vi "FPGA_ADC_test.vi"() -> ()   [LabVIEW 2013]
uses:
  <vilib>/rvi/interface/nirviReadWriteControl/nirviReadWriteControl.xnode
  fpga-bitfile-ref.ctl
  <vilib>/rvi/interface/nirviCloseFPGA/nirviCloseFPGA.xnode
  FPGA Bitfiles/fpgabatch18_sbRIO9612RIO0_FPGAMAINlock-in_BbNldMosBaM.lvbitx
  <vilib>/rvi/errors/niLvFpgaMergeErrorWithErrorCode.vi
  <vilib>/rvi/errors/niLvFpgaAdjustHostInterfaceError.vi
  <vilib>/FPGAPlugInAG/sbRIO-9612/niLvFpga_Close_sbRIO-9612.vi
panel:
  out "data out":dbl[][](array[numeric])
  out "output cluster 2":T1
  out "output cluster":T2={"trig mode"=enum."ramp", "Nchannels"=0, "Navg"=0, "trig edge"=enum."falling", "trig input"=0, "Npts to read"=0, "Nchannels"=0, "clock divider"=0, "Data [i]"=0.0, "Configurations"=[0, 0, 0, 0, 0, 0, 0, 0, 0, 0, 0, 0, 0, 0, 0, 0, 0, 0, 0, 0, 0, 0, 0, 0, 0, 0, 0, 0, 0, 0, 0, 0]}
  in  "IP Address":string="192.168.137.11"
  in  "Inst_parameter":T3={"Kind"=17, "Strings"=["ADC", "192.168.137.11", "V0;V1", "V;V", "1.0;1.0", "0;1", "10;10", "RSE;RSE"], "uint64s"=[2, 250000, 1, 1, 0, 0, 1], "Doubles"=[1.0], "DAQmx take out list"=[]}
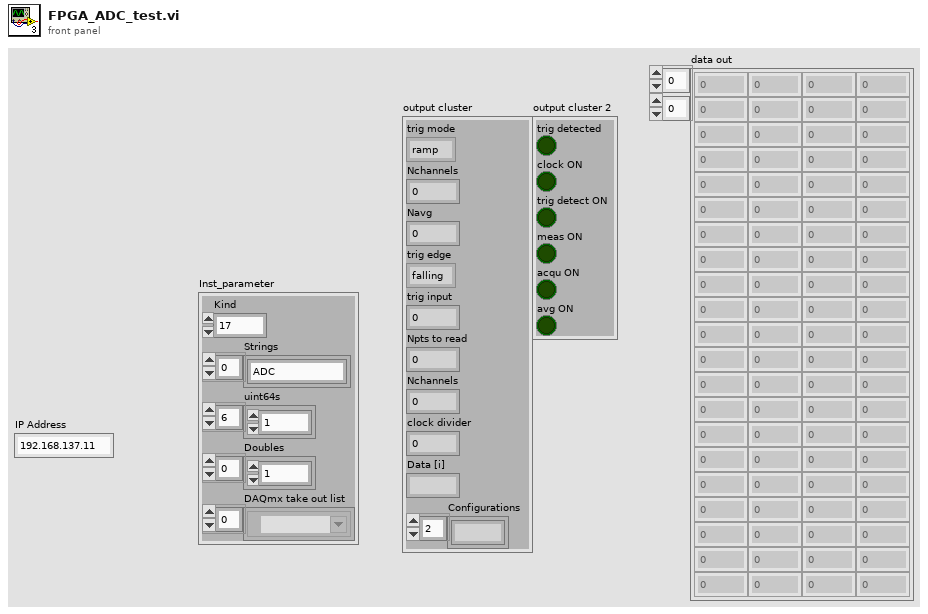
[diagram p1: front panel]
types:
  T1 = cluster{"trig detected":bool, "clock ON":bool, "trig detect ON":bool, "meas ON":bool, "acqu ON":bool, "avg ON":bool}
  T2 = cluster{"trig mode":enum16{"ramp", "RT"}, "Nchannels":i32, "Navg":u32, "trig edge":enum16{"falling", "rising", "both"}, "trig input":i16, "Npts to read":i16, "Nchannels":i32, "clock divider":u32, "Data [i]":fxp<+/-,26,5>, "Configurations":u16[]}
  T3 = cluster{"Kind":u16, "Strings":string[], "uint64s":u64[], "Doubles":dbl[], "DAQmx take out list":refnum<k21>[]}
  T4 = typedef "fpga-bitfile-ref.ctl" = refnum<k20>
  T5 = cluster{"trig detected":void, "clock ON":void, "trig detect ON":void, "meas ON":void, "acqu ON":void, "avg ON":void}
  T6 = cluster{"trig mode":void, "Nchannels":void, "Navg":void, "trig edge":void, "trig input":void, "Npts to read":void, "Nchannels":void, "clock divider":void, "Data [i]":void, "Configurations":void}
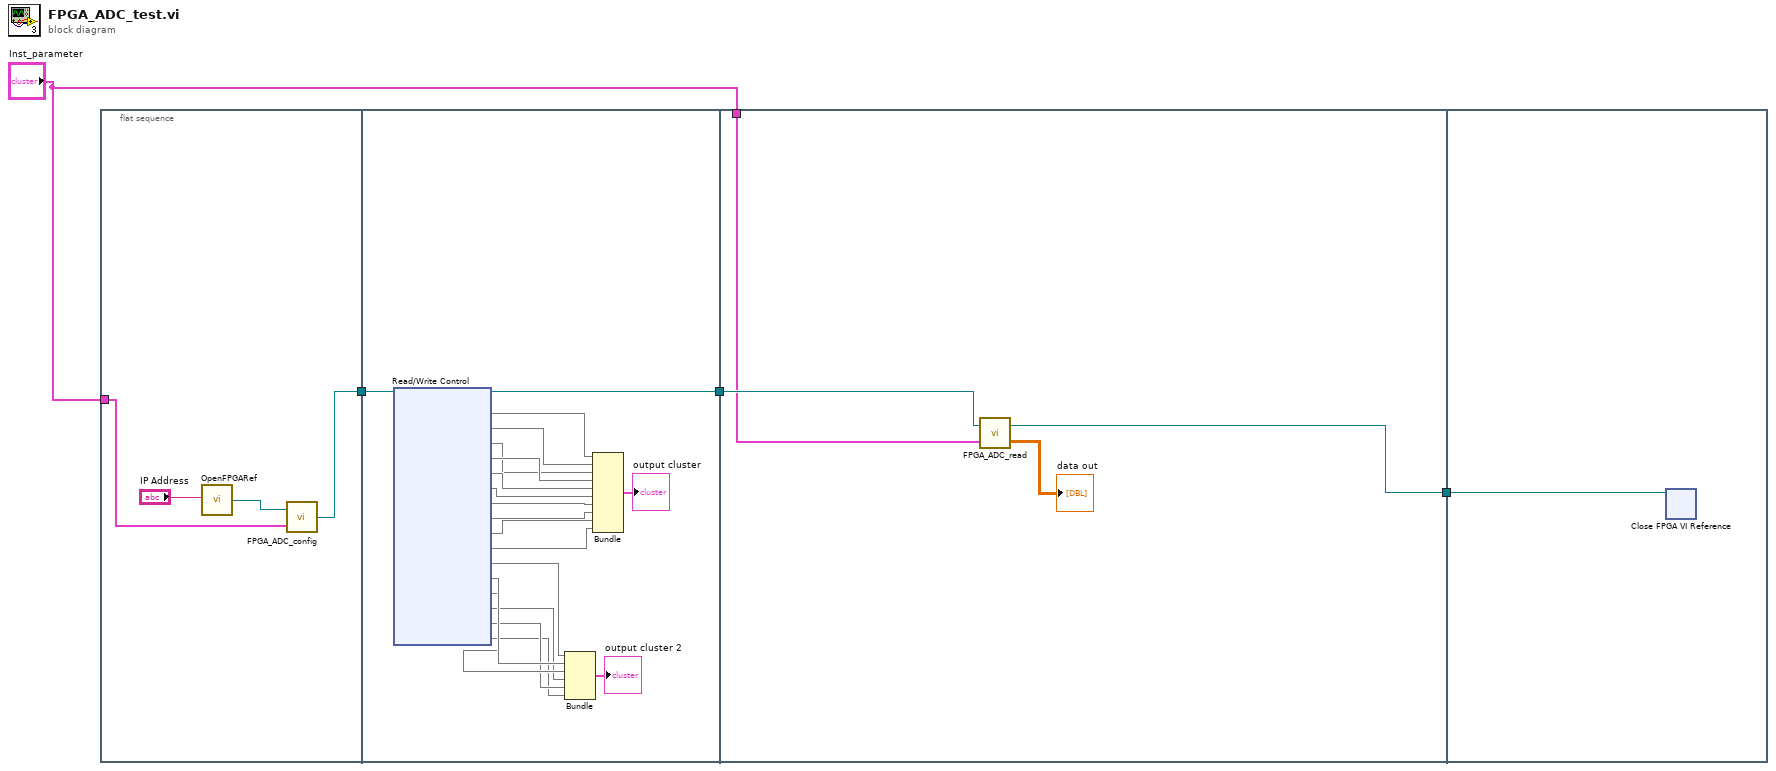
[diagram p0: block diagram]
diagram:
  n1 = flat-sequence {
    tunnel: "Inst_parameter" -> [w5]
    tunnel: [w6] -> w4
    tunnel: w4 -> [w28]
    tunnel: [w27] -> w3
    tunnel: w3 -> [w30]
    tunnel: "Inst_parameter" -> [w29]
    tunnel: [w31] -> w1
    tunnel: w1 -> [w33]
    frame #0 {
      n2 = call "OpenFPGARef.vi"("IP Address"="IP Address") -> ("FPGA VI Reference Out"=w7:T4)
      n3 = call "FPGA_ADC_config.vi"("Inst_parameter"=w5, "FPGA ref in"=w7) -> ("FPGA ref out"=w6:T4)
    }
    frame #1 {
      n4 = xnode "Read/Write Control"("FPGA VI Reference In"=w28) -> ("FPGA VI Reference Out"=w27:T4, "trig mode"=w18, "Nchannels"=w19, "Navg"=w20, "trig edge"=w21, "trig input"=w22, "Npts to read"=w23, "Nchannels"=w24, "clock divider"=w25, "Data [i]"=w26, "Configurations"=w11, "trig detected"=w17, "clock ON"=w16, "trig detect ON"=w15, "meas ON"=w14, "acqu ON"=w13, "avg ON"=w12)  [unwired: 1 in, 1 out]
      n5 = Bundle("trig detected"=w17, "clock ON"=w16, "trig detect ON"=w15, "meas ON"=w14, "acqu ON"=w13, "avg ON"=w12) -> (→"output cluster 2":T5)  [unwired: 1 in]
      n6 = Bundle("trig mode"=w18, "Nchannels"=w19, "Navg"=w20, "trig edge"=w21, "trig input"=w22, "Npts to read"=w23, "Nchannels"=w24, "clock divider"=w25, "Data [i]"=w26, "Configurations"=w11) -> (→"output cluster":T6)  [unwired: 1 in]
    }
    frame #2 {
      n7 = call "FPGA_ADC_read.vi"("Readout parameter"=w29, "FPGA In"=w30) -> ("data out"=→"data out":dbl[][], "FPGA Out"=w31:T4)
    }
    frame #3 {
      n8 = xnode "Close FPGA VI Reference"("FPGA VI Reference In"=w33) -> ()  [unwired: 1 in, 1 out]
    }
  }
